vi "Teleop.vi"(10 "Match Info":T1={"Autonomous Elapsed Seconds"=0.0, "TeleOp Elapsed Seconds"=0.0, "Disabled Elapsed Seconds"=0.0, "Visited Autonomous"=FALSE, "Visited TeleOp"=FALSE, "Visited Disabled"=FALSE, "Autonomous Settings"={"Autonomous Style"=enum."Independent", "VI Refnum"=refnum}}, 11 "Call Context":T2) -> ()   [LabVIEW 2014]
doc: "This VI is called for each TeleOp packet received from the DS where the robot is not disabled. It is often used to read from the joysticks and update I/O or to update setpoints for timed control loops. It should complete and return within 20 milliseconds or it may miss DS packets."
uses:
  <vilib>/Rock Robotics/WPI/DriverStation/WPI_DriverStationDerivedRobotMode.ctl
  <vilib>/Rock Robotics/WPI/DriverStation/WPI_DriverStationMatch Info.ctl
  <vilib>/Rock Robotics/WPI/RobotDrive/WPI_RobotDriveGetSetRefNum.vi
  <vilib>/Rock Robotics/WPI/Joystick/WPI_JoystickGetSetRefNum.vi
  <vilib>/Rock Robotics/Network Tables/SD Write Boolean Array.vi
  <vilib>/Rock Robotics/Network Tables/SD Write Numeric Array.vi
  <vilib>/Rock Robotics/Network Tables/SD Read Boolean.vi
  <vilib>/Rock Robotics/Network Tables/SD Read Number.vi
  Robot Global Data.vi
panel:
  out "Switch Pressed 2":bool
  out "Elevator Encoder Ticks":dbl
  out "Encoder Ticks":dbl
  out "Encoder Ticks":dbl
  out "Sample Slider 0":dbl(slide) scale=0.0..5.0
  out "Sample Boolean 1":bool
  out "Sample Boolean 0":bool
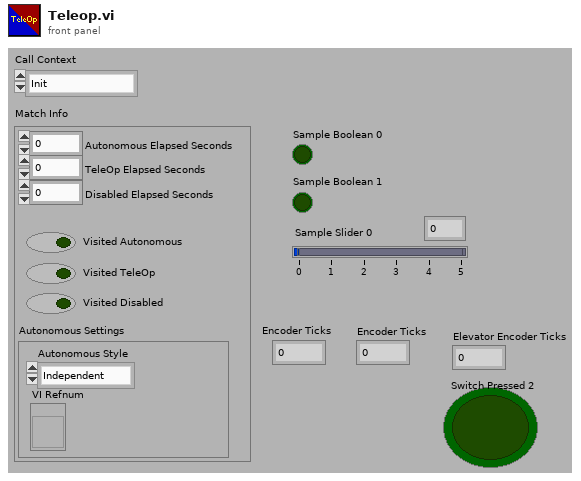
[diagram p1: front panel]
types:
  T1 = typedef "WPI_DriverStationMatch Info.ctl" = cluster{"Autonomous Elapsed Seconds":dbl, "TeleOp Elapsed Seconds":dbl, "Disabled Elapsed Seconds":dbl, "Visited Autonomous":bool, "Visited TeleOp":bool, "Visited Disabled":bool, "Autonomous Settings":cluster{"Autonomous Style":enum16{"Iterative", "Independent"}, "VI Refnum":refnum<vi>}}
  T2 = typedef "WPI_DriverStationDerivedRobotMode.ctl" = enum16{"Init", "Execute", "Stop"}
  T3 = typedef "WPI_RobotDriveDevRef.ctl" = cluster{"DevStatus":errorcluster, "Motors[]":T4[], "Square Inputs":bool, "Max Output":dbl}
  T4 = typedef "WPI_MotorControlDeviceRef.ctl" = cluster{"DeviceStatus":errorcluster, "Type":T5, "PWM":cluster{"Controller":T6, "PWM Channel":T7, "DeadBand":T8}, "CAN":cluster{"Device Number":u8, "Control Mode":T9, "Semaphore":T10, "Max Vout":dbl, "TalonSRX Control Mode":T11}, "Invert":bool, "TransformRef":T12, "InvTransformRef":T12}
  T5 = typedef "WPI_MotorControlType.ctl" = enum16{"PWM", "CAN", "CANTalonSRX"}
  T6 = typedef "FPGA_TypedefDigitalModule.ctl" = enum16{"Controller 1"}
  T7 = typedef "FPGA_DIOPWMChannel.ctl" = enum8{"PWM 0", "PWM 1", "PWM 2", "PWM 3", "PWM 4", "PWM 5", "PWM 6", "PWM 7", "PWM 8", "PWM 9", "PWM MXP 0", "PWM MXP 1", "PWM MXP 2", "PWM MXP 3", "PWM MXP 4", "PWM MXP 5", "PWM MXP 6", "PWM MXP 7", "PWM MXP 8", "PWM MXP 9", "Invalid"}
  T8 = typedef "WPI_PWMDeadband.ctl" = cluster{"Name":string, "maxPositivePwm":i32, "minPositivePwm":i32, "centerPwm":i32, "maxNegativePwm":i32, "minNegativePwm":i32, "angularRange":u16}
  T9 = typedef "WPI_CANJaguar_ControlMode.ctl" = enum8{"Percent VBus", "Current", "Speed", "Position", "Voltage"}
  T10 = typedef "Semaphore RefNum" = refnum<k1>
  T11 = typedef "WPI_CANTalonSRX_APIControlMode.ctl" = enum8{"Percent VBus", "Speed", "Position", "Slave", "Unchanged / Invalid"}
  T12 = typedef "WPI_PWMTransform_ConPane.ctl" = refnum<vi>
  T13 = typedef "WPI_JoystickDevRef.ctl" = cluster{"Device":T14}
  T14 = typedef "WPI_JoystickDeviceEnum.ctl" = enum16{"USB 0", "USB 1", "USB 2", "USB 3", "USB 4", "USB 5"}
  T15 = typedef "WPI_EncoderDevRef.ctl" = cluster{"DevStatus":errorcluster, "EncoderIndex":T16, "CounterIndex":T17, "DistancePerCount":dbl, "Decoding Type":T18}
  T16 = typedef "FPGA_EncoderIdx.ctl" = enum8{"Enc 0", "Enc 1", "Enc 2", "Enc 3", "Enc 4", "Enc 5", "Enc 6", "Enc 7", "Invalid"}
  T17 = typedef "FPGA_CounterCtrSystemIndex.ctl" = enum8{"Ctr 0", "Ctr 1", "Ctr 2", "Ctr 3", "Ctr 4", "Ctr 5", "Ctr 6", "Ctr 7", "Invalid"}
  T18 = typedef "WPI_EncoderType.ctl" = enum16{"1x", "2x", "4x"}
  T19 = typedef "WPI_SwitchDevRef.ctl" = cluster{"DevStatus":errorcluster, "DIO Channel":T20, "Controller":T6, "CntIndex":T17, "Normally Closed":bool}
  T20 = typedef "FPGA_DIOChannel.ctl" = enum8{"DIO 0", "DIO 1", "DIO 2", "DIO 3", "DIO 4", "DIO 5", "DIO 6", "DIO 7", "DIO 8", "DIO 9", "DIO MXP 0", "DIO MXP 1", "DIO MXP 2", "DIO MXP 3", "DIO MXP 4", "DIO MXP 5", "DIO MXP 6", "DIO MXP 7", "DIO MXP 8", "DIO MXP 9", "DIO MXP 10", "DIO MXP 11", "DIO MXP 12", "DIO MXP 13", "DIO MXP 14", "DIO MXP 15", "Invalid"}
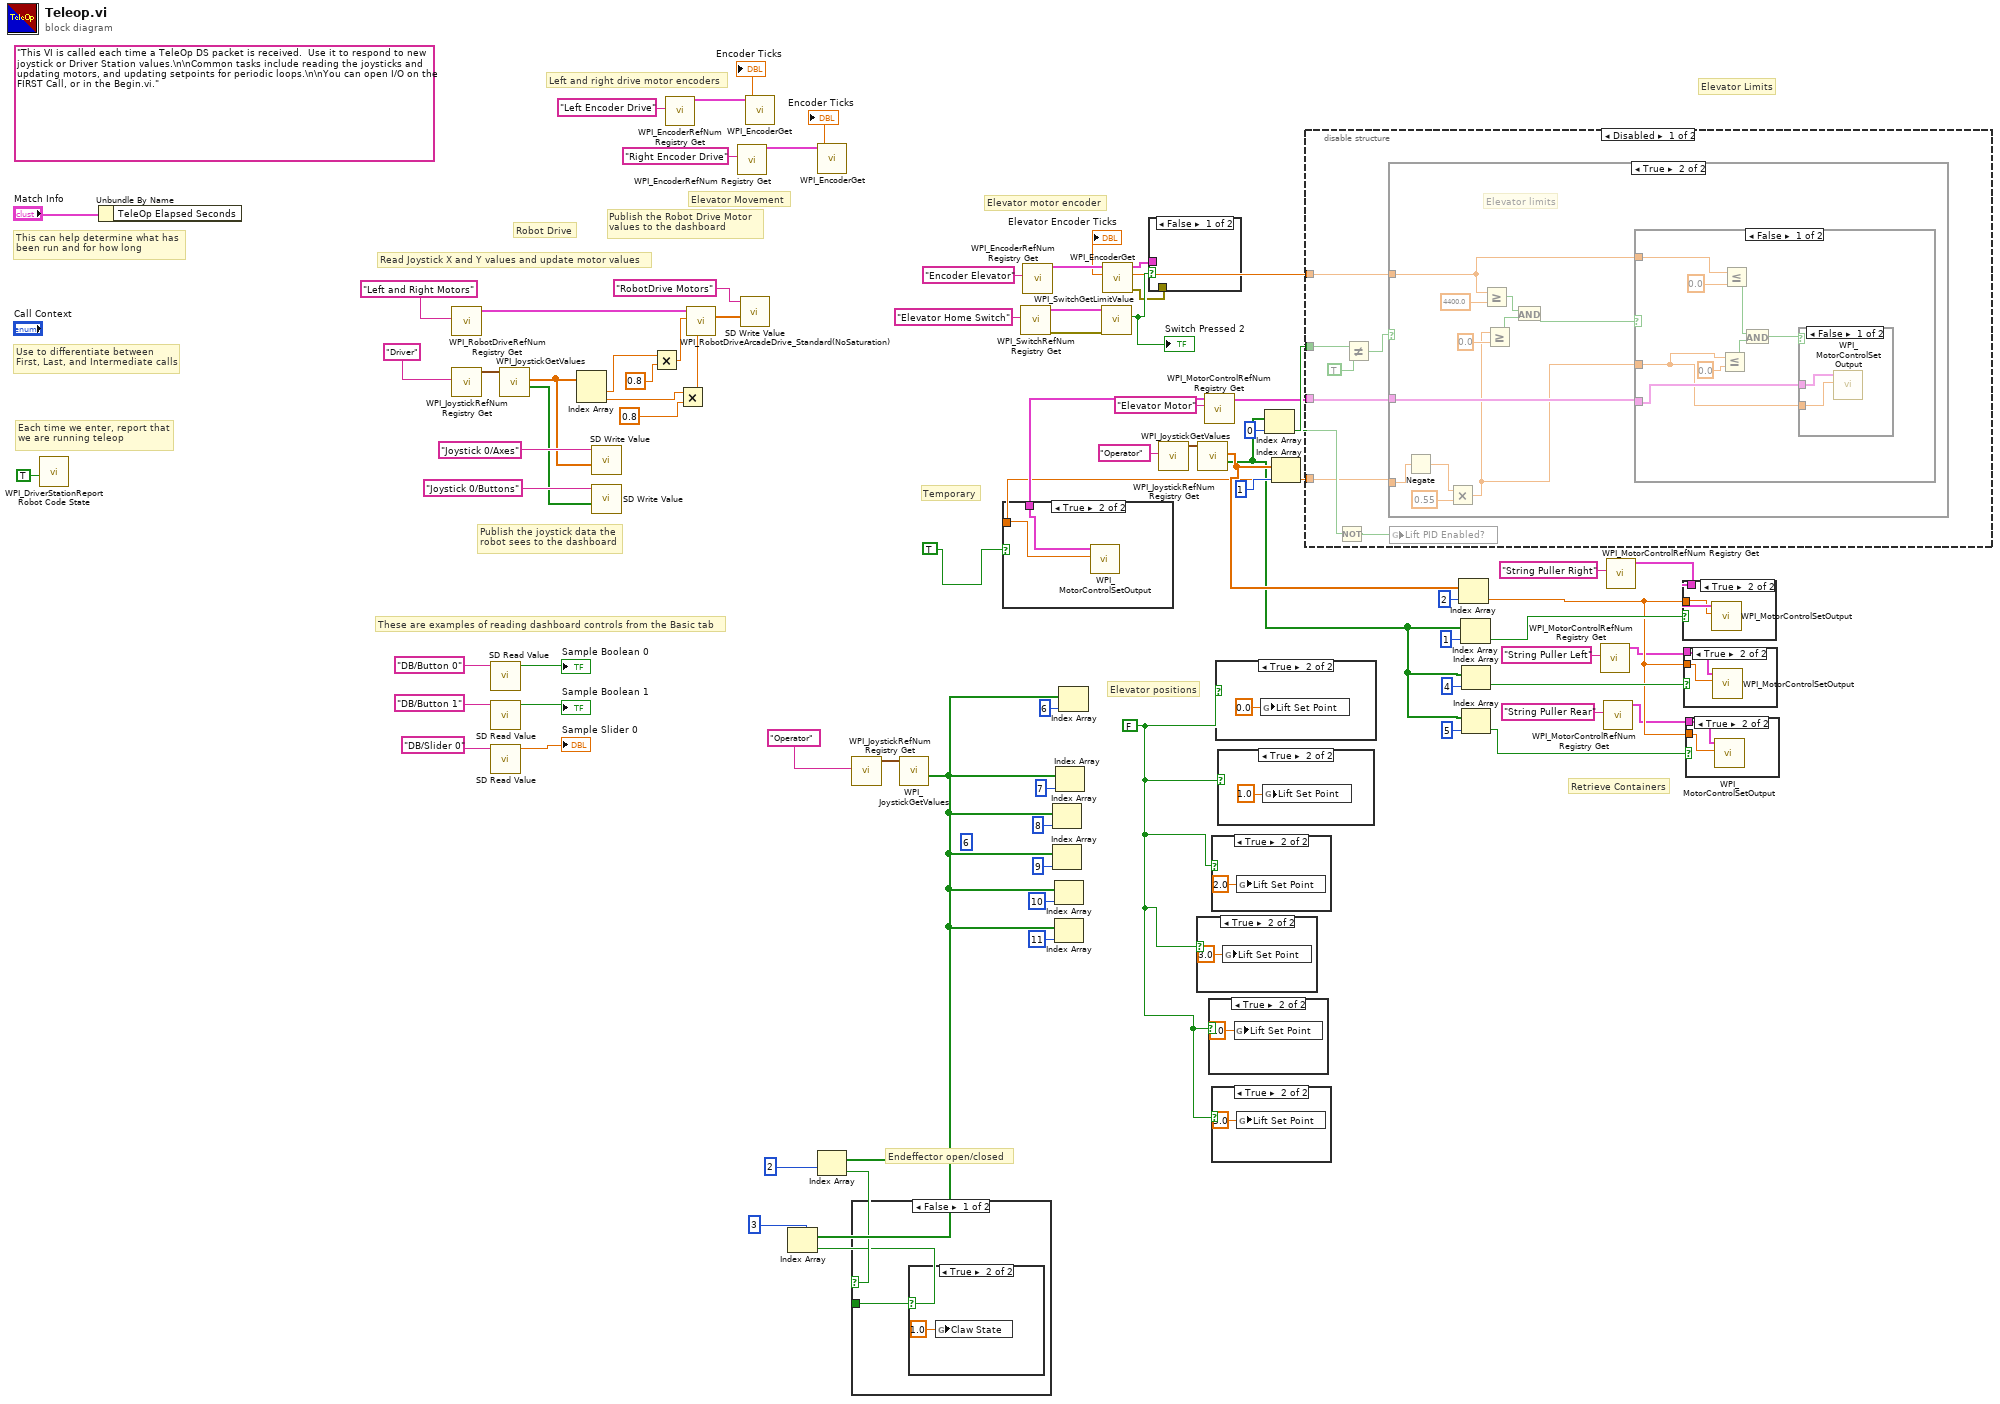
[diagram p0: block diagram]
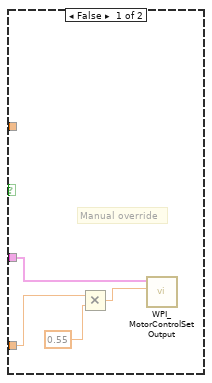
[diagram p2: hidden frame]
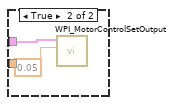
[diagram p3: hidden frame]
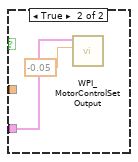
[diagram p4: hidden frame]
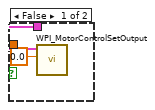
[diagram p6: hidden frame]
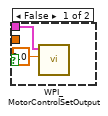
[diagram p7: hidden frame]
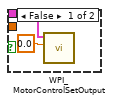
[diagram p8: hidden frame]
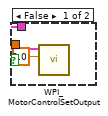
[diagram p9: hidden frame]
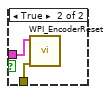
[diagram p10: hidden frame]
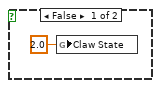
[diagram p11: hidden frame]
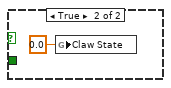
[diagram p12: hidden frame]
diagram:
  w2 = FALSE
  (unwired) 6 ("index")
  (unwired) "This VI is called each time a TeleOp DS packet is received.  Use it to respond to new joystick or Driver Station values.\n\nCommon tasks include reading the joysticks and updating motors, and updating setpoints for periodic loops.\n\nYou can open I/O on the FIRST Call, or in the Begin.vi."
  # "Temporary"
  # "Retrieve Containers"
  # "Elevator Limits"
  # "Endeffector open/closed"
  # "Elevator positions"
  # "Elevator motor encoder"
  # "Left and right drive motor encoders"
  # "Robot Drive"
  # "Elevator Movement"
  # "These are examples of reading dashboard controls from the Basic tab"
  # "Publish the Robot Drive Motor\nvalues to the dashboard"
  # "Publish the joystick data the\nrobot sees to the dashboard"
  # "Each time we enter, report that\nwe are running teleop"
  # "Use to differentiate between\nFirst, Last, and Intermediate calls"
  # "This can help determine what has\nbeen run and for how long"
  # "Read Joystick X and Y values and update motor values"
  n1 = call <vilib>:"WPI_DriverStationReport Robot Code State.vi"("TeleOp"=TRUE ("Autonomous")) -> ()  [unwired: 10 in, 1 out]
  n2 = Unbundle By Name("Match Info") -> ()  [unwired: 1 out]
  n3 = call <vilib>:"WPI_RobotDriveRefNum Registry Get.vi"("refnum name"="Left and Right Motors") -> ("RobotDriveDevRef"=w76:T3)  [unwired: 1 in, 9 out]
  n4 = call <vilib>:"WPI_JoystickRefNum Registry Get.vi"("refnum name"="Driver") -> ("JoystickDevRef"=w74:T13)  [unwired: 1 in, 9 out]
  n5 = call-poly <vilib>:"SD Read Value.vi"("Name"="DB/Button 0" ("refnum name")) -> ("Boolean"=→"Sample Boolean 0":bool)  [unwired: 8 in, 2 out]
  n6 = call-poly <vilib>:"SD Read Value.vi"("Name"="DB/Button 1" ("refnum name")) -> ("Boolean"=→"Sample Boolean 1":bool)  [unwired: 8 in, 2 out]
  n7 = call-poly <vilib>:"SD Read Value.vi"("Name"="DB/Slider 0" ("refnum name")) -> ("Numeric"=→"Sample Slider 0":dbl)  [unwired: 8 in, 2 out]
  n8 = call <vilib>:"WPI_JoystickGetValues.vi"("JoystickDevRef"=w74) -> ("Buttons"=w61:bool[], "Axes"=w63:dbl[])  [unwired: 6 in, 3 out]
  n9 = Index Array(array=w63) -> (element #1=w19:dbl, element #2=w22:dbl)  [unwired: 2 in]
  n10 = call-poly <vilib>:"SD Write Value.vi"("Numeric Array"=w63, "Name"="Joystick 0/Axes") -> ()  [unwired: 8 in, 2 out]
  n11 = call-poly <vilib>:"SD Write Value.vi"("Boolean Array"=w61, "Name"="Joystick 0/Buttons") -> ()  [unwired: 8 in, 2 out]
  n12 = Multiply(x=w19, y=0.8) -> (x*y=w21:dbl)
  n13 = call <vilib>:"WPI_EncoderRefNum Registry Get.vi"("refnum name"="Left Encoder Drive") -> ("EncoderDevRef"=w43:T15)  [unwired: 9 in, 1 out]
  n14 = Multiply(x=w22, y=0.8) -> (x*y=w24:dbl)
  n15 = call <vilib>:"WPI_RobotDriveArcadeDrive_Standard(NoSaturation).vi"("Y axis value"=w24, "X axis value"=w21, "RobotDriveDevRef"=w76) -> ("Motor Values"=w65:dbl[])  [unwired: 1 in, 7 out]
  n16 = call <vilib>:"WPI_EncoderRefNum Registry Get.vi"("refnum name"="Right Encoder Drive") -> ("EncoderDevRef"=w46:T15)  [unwired: 9 in, 1 out]
  n17 = call-poly <vilib>:"SD Write Value.vi"("Numeric Array"=w65, "Name"="RobotDrive Motors") -> ()  [unwired: 8 in, 2 out]
  n18 = call <vilib>:"WPI_EncoderGet.vi"("EncoderDevRef"=w43) -> ("Distance"=→"Encoder Ticks":dbl)  [unwired: 5 in, 5 out]
  n19 = call <vilib>:"WPI_EncoderGet.vi"("EncoderDevRef"=w46) -> ("Distance"=→"Encoder Ticks":dbl)  [unwired: 5 in, 5 out]
  n20 = call <vilib>:"WPI_JoystickRefNum Registry Get.vi"("refnum name"="Operator") -> ("JoystickDevRef"=w60:T13)  [unwired: 1 in, 9 out]
  n21 = call <vilib>:"WPI_JoystickGetValues.vi"("JoystickDevRef"=w60) -> ("Buttons"=w50:bool[])  [unwired: 6 in, 4 out]
  n22 = Index Array(array=w50, index=3) -> (element=w48:bool)
  n23 = Index Array(array=w50, index=2) -> (element=w49:bool)
  n24 = case shown="False" w49 {
    tunnel: w48 -> [w79 _]
    frame False {
      n25 = case shown="True" w79 {
        frame False {
          n26 = global write "Robot Global Data.vi" "Claw State"(2.0 ("Claw State")) -> ()
        }
        frame True {
          n27 = global write "Robot Global Data.vi" "Claw State"(1.0 ("Claw State")) -> ()
        }
      }
    }
    frame True {
      n28 = global write "Robot Global Data.vi" "Claw State"(0.0 ("Claw State")) -> ()
    }
  }
  n29 = call <vilib>:"WPI_SwitchRefNum Registry Get.vi"("refnum name"="Elevator Home Switch") -> ("error out"=w37:errorcluster, "SwitchDevRef"=w38:T19)  [unwired: 9 in]
  n30 = call <vilib>:"WPI_EncoderRefNum Registry Get.vi"("refnum name"="Encoder Elevator") -> ("EncoderDevRef"=w40:T15)  [unwired: 9 in, 1 out]
  n31 = Index Array(array=w50, index=8) -> ()  [unwired: 1 out]
  n32 = Index Array(array=w50, index=9) -> ()  [unwired: 1 out]
  n33 = Index Array(array=w50, index=10) -> ()  [unwired: 1 out]
  n34 = Index Array(array=w50, index=11) -> ()  [unwired: 1 out]
  n35 = Index Array(array=w50, index=7) -> ()  [unwired: 1 out]
  n36 = Index Array(array=w50, index=6) -> ()  [unwired: 1 out]
  n37 = call <vilib>:"WPI_SwitchGetLimitValue.vi"("error in (no error)"=w37, "SwitchDevRef"=w38) -> ("Switch Pressed"=w36:bool)  [unwired: 7 in, 2 out]
  "Switch Pressed 2" <- w36
  n38 = call <vilib>:"WPI_EncoderGet.vi"("EncoderDevRef"=w40) -> ("error out"=w34:errorcluster, "Distance"=w29:dbl, "EncoderDevRef"=w35:T15)  [unwired: 5 in, 3 out]
  "Elevator Encoder Ticks" <- w29
  n39 = case shown="False" w36 {
    tunnel: w35 -> [_ w84]
    tunnel: w34 -> [_ w83]
    frame False {
    }
    frame True {
      n40 = call <vilib>:"WPI_EncoderReset.vi"("error in (no error)"=w83, "EncoderDevRef"=w84) -> ()  [unwired: 8 in, 2 out]
    }
  }
  n41 = call <vilib>:"WPI_JoystickRefNum Registry Get.vi"("refnum name"="Operator") -> ("JoystickDevRef"=w31:T13)  [unwired: 9 in, 1 out]
  n42 = case shown="True" w2 {
    frame False {
    }
    frame True {
      n43 = global write "Robot Global Data.vi" "Lift Set Point"(3.0 ("Lift Set Point")) -> ()
    }
  }
  n44 = call <vilib>:"WPI_JoystickGetValues.vi"("JoystickDevRef"=w31) -> ("Buttons"=w25:bool[], "Axes"=w26:dbl[])  [unwired: 6 in, 3 out]
  n45 = call <vilib>:"WPI_MotorControlRefNum Registry Get.vi"("refnum name"="Elevator Motor") -> ("MotorControlDevRef"=w4:T4)  [unwired: 9 in, 1 out]
  n46 = case shown="True" w2 {
    frame False {
    }
    frame True {
      n47 = global write "Robot Global Data.vi" "Lift Set Point"(4.0 ("Lift Set Point")) -> ()
    }
  }
  n48 = case shown="True" w2 {
    frame False {
    }
    frame True {
      n49 = global write "Robot Global Data.vi" "Lift Set Point"(2.0 ("Lift Set Point")) -> ()
    }
  }
  n50 = case shown="True" w2 {
    frame False {
    }
    frame True {
      n51 = global write "Robot Global Data.vi" "Lift Set Point"(5.0 ("Lift Set Point")) -> ()
    }
  }
  n52 = case shown="True" w2 {
    frame False {
    }
    frame True {
      n53 = global write "Robot Global Data.vi" "Lift Set Point"(0.0 ("Lift Set Point")) -> ()
    }
  }
  n54 = case shown="True" w2 {
    frame False {
    }
    frame True {
      n55 = global write "Robot Global Data.vi" "Lift Set Point"(1.0 ("Lift Set Point")) -> ()
    }
  }
  n56 = Index Array(array=w25, index=0) -> (element=w27:bool)
  n57 = Index Array(array=w26, index=1) -> (element=w3:dbl)
  n58 = case shown="True" TRUE {
    tunnel: w3 -> [_ w94]
    tunnel: w4 -> [w92 w93]
    frame False {
      n59 = call <vilib>:"WPI_MotorControlSetOutput.vi"("Output"=0.0, "MotorControlDevRef"=w92) -> ()  [unwired: 7 in, 3 out]
    }
    frame True {
      n60 = call <vilib>:"WPI_MotorControlSetOutput.vi"("Output"=w94, "MotorControlDevRef"=w93) -> ()  [unwired: 7 in, 3 out]
    }
  }
  n61 = disable-structure shown="Disabled" {
    disable-tunnel: w29 -> [w101 _]
    disable-tunnel: w27 -> [w99 _]
    disable-tunnel: w4 -> [w97 _]
    disable-tunnel: w3 -> [w96 _]
    frame Disabled {
      n62 = Not(x=w99) -> (.not. x?=w98:bool)
      n63 = Not Equal?(x=w99, y=TRUE) -> (x != y?=w95:bool)
      n64 = case shown="True" w95 {
        tunnel: w97 -> [w105 w111]
        tunnel: w96 -> [w103 w110]
        tunnel: w101 -> [_ w106]
        frame False {
          # "Manual override"
          n65 = Multiply(x=w103, y=0.55) -> (x*y=w102:dbl)
          n66 = call <vilib>:"WPI_MotorControlSetOutput.vi"("Output"=w102, "MotorControlDevRef"=w105) -> ()  [unwired: 7 in, 3 out]
        }
        frame True {
          # "Elevator limits"
          n67 = Negate(x=w110) -> (-x=w109:dbl)
          n68 = Multiply(x=w109, y=0.55) -> (x*y=w107:dbl)
          n69 = Greater Or Equal?(x=w106, y=4400.0) -> (x >= y?=w113:bool)
          n70 = Greater Or Equal?(x=w107, y=0.0) -> (x >= y?=w114:bool)
          n71 = And(x=w113, y=w114) -> (x .and. y?=w112:bool)
          n72 = case shown="False" w112 {
            tunnel: w111 -> [w118 w130]
            tunnel: w107 -> [w117 _]
            tunnel: w106 -> [w124 _]
            frame False {
              n73 = Less Or Equal?(x=w117, y=0.0) -> (x <= y?=w120:bool)
              n74 = Less Or Equal?(x=w124, y=0.0) -> (x <= y?=w121:bool)
              n75 = And(x=w121, y=w120) -> (x .and. y?=w119:bool)
              n76 = case shown="False" w119 {
                tunnel: w118 -> [w126 w128]
                tunnel: w117 -> [w125 _]
                frame False {
                  n77 = call <vilib>:"WPI_MotorControlSetOutput.vi"("Output"=w125, "MotorControlDevRef"=w126) -> ()  [unwired: 7 in, 3 out]
                }
                frame True {
                  n78 = call <vilib>:"WPI_MotorControlSetOutput.vi"("Output"=0.05, "MotorControlDevRef"=w128) -> ()  [unwired: 7 in, 3 out]
                }
              }
            }
            frame True {
              n79 = call <vilib>:"WPI_MotorControlSetOutput.vi"("Output"=-0.05, "MotorControlDevRef"=w130) -> ()  [unwired: 7 in, 3 out]
            }
          }
        }
      }
      n80 = global write "Robot Global Data.vi" "Lift PID Enabled?"(w98) -> ()
    }
    frame Enabled {
    }
  }
  n81 = Index Array(array=w26, index=2) -> (element=w9:dbl)
  n82 = Index Array(array=w25, index=1) -> (element=w14:bool)
  n83 = Index Array(array=w25, index=4) -> (element=w11:bool)
  n84 = Index Array(array=w25, index=5) -> (element=w10:bool)
  n85 = call <vilib>:"WPI_MotorControlRefNum Registry Get.vi"("refnum name"="String Puller Left") -> ("MotorControlDevRef"=w6:T4)  [unwired: 9 in, 1 out]
  n86 = call <vilib>:"WPI_MotorControlRefNum Registry Get.vi"("refnum name"="String Puller Rear") -> ("MotorControlDevRef"=w5:T4)  [unwired: 9 in, 1 out]
  n87 = call <vilib>:"WPI_MotorControlRefNum Registry Get.vi"("refnum name"="String Puller Right") -> ("MotorControlDevRef"=w12:T4)  [unwired: 9 in, 1 out]
  n88 = case shown="True" w14 {
    tunnel: w9 -> [_ w133]
    tunnel: w12 -> [w132 w134]
    frame False {
      n89 = call <vilib>:"WPI_MotorControlSetOutput.vi"("Output"=0.0, "MotorControlDevRef"=w132) -> ()  [unwired: 7 in, 3 out]
    }
    frame True {
      n90 = call <vilib>:"WPI_MotorControlSetOutput.vi"("Output"=w133, "MotorControlDevRef"=w134) -> ()  [unwired: 7 in, 3 out]
    }
  }
  n91 = case shown="True" w11 {
    tunnel: w9 -> [_ w138]
    tunnel: w6 -> [w135 w137]
    frame False {
      n92 = call <vilib>:"WPI_MotorControlSetOutput.vi"("Output"=0.0, "MotorControlDevRef"=w135) -> ()  [unwired: 7 in, 3 out]
    }
    frame True {
      n93 = call <vilib>:"WPI_MotorControlSetOutput.vi"("Output"=w138, "MotorControlDevRef"=w137) -> ()  [unwired: 7 in, 3 out]
    }
  }
  n94 = case shown="True" w10 {
    tunnel: w9 -> [_ w142]
    tunnel: w5 -> [w139 w141]
    frame False {
      n95 = call <vilib>:"WPI_MotorControlSetOutput.vi"("Output"=0.0, "MotorControlDevRef"=w139) -> ()  [unwired: 7 in, 3 out]
    }
    frame True {
      n96 = call <vilib>:"WPI_MotorControlSetOutput.vi"("Output"=w142, "MotorControlDevRef"=w141) -> ()  [unwired: 7 in, 3 out]
    }
  }
